vi "calibrateSteps.vi"(8 "error out":errorcluster, 9 "Direction":dbl, 10 "controllerAddress":i32, 11 "reference out":refnum<k24>) -> (0 "error out 2":errorcluster, 1 "mmPerStep":dbl, 2 "controllerAddress out":i32, 3 "reference out 2":refnum<k24>)   [LabVIEW 2013]
uses:
  C:/Program Files/Newport/Piezo Motion Control/Newport AG-UC2-UC8 Applet/Samples/LabVIEW 2009/AgilisCmdLib.dll
  Program Files/Newport/Piezo Motion Control/Newport AG-UC2-UC8 Applet/Samples/LabVIEW 2009/AgilisCmdLib.dll
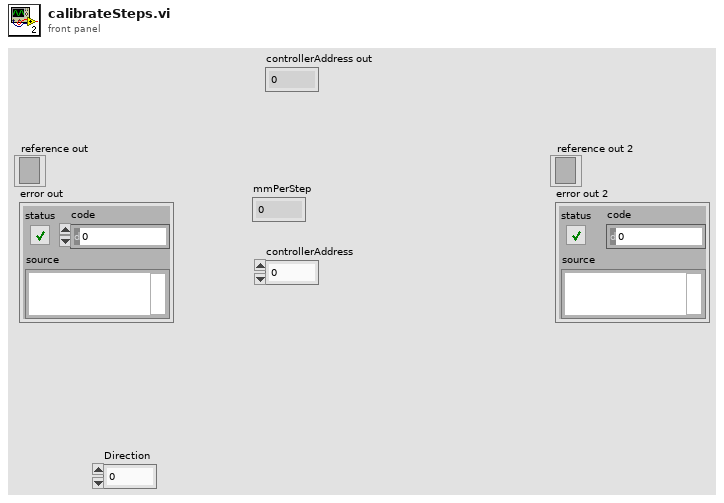
[diagram p1: front panel]
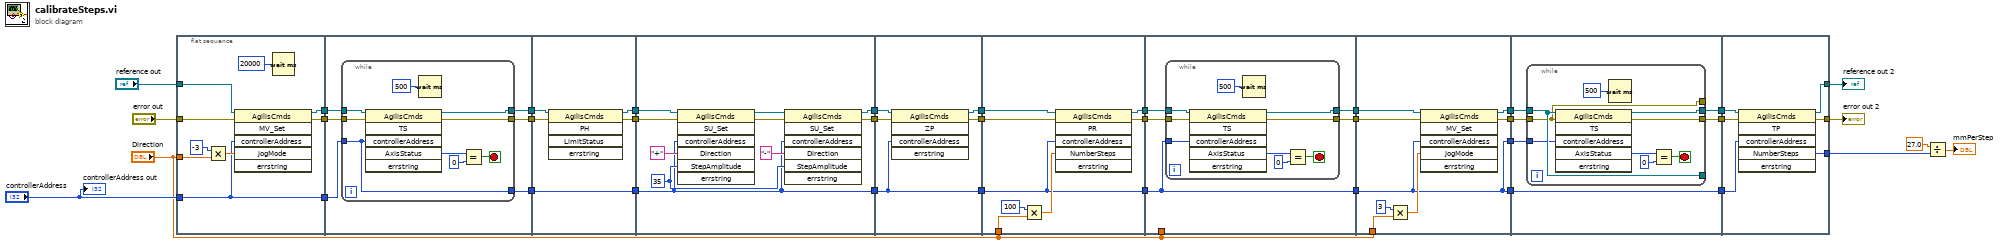
[diagram p0: block diagram]
diagram:
  n1 = flat-sequence {
    tunnel: "Direction" -> [w39]
    tunnel: "controllerAddress" -> [w40]
    tunnel: "error out" -> [w43]
    tunnel: "reference out" -> [w44]
    tunnel: [w42] -> w21
    tunnel: [w41] -> w20
    tunnel: [w40] -> w17
    tunnel: [w52] -> w37
    tunnel: [w51] -> w36
    tunnel: w21 -> [w50]
    tunnel: w20 -> [w49]
    tunnel: w17 -> [w48]
    tunnel: [w47] -> w15
    tunnel: w37 -> [w66]
    tunnel: w36 -> [w63]
    tunnel: [w65] -> w35
    tunnel: [w64] -> w34
    tunnel: [w62] -> w16
    tunnel: w15 -> [w62]
    tunnel: w35 -> [w75]
    tunnel: w34 -> [w74]
    tunnel: [w70] -> w33
    tunnel: [w72] -> w32
    tunnel: w16 -> [w67]
    tunnel: [w67] -> w14
    tunnel: w33 -> [w81]
    tunnel: w32 -> [w80]
    tunnel: [w79] -> w19
    tunnel: [w78] -> w18
    tunnel: w14 -> [w77]
    tunnel: [w77] -> w13
    tunnel: w19 -> [w87]
    tunnel: w18 -> [w86]
    tunnel: w13 -> [w85]
    tunnel: [w85] -> w12
    tunnel: [w84] -> w11
    tunnel: [w83] -> w10
    tunnel: "Direction" -> [w82]
    tunnel: [w94] -> w31
    tunnel: [w93] -> w30
    tunnel: "Direction" -> [_]
    tunnel: w12 -> [w90]
    tunnel: w11 -> [w92]
    tunnel: w10 -> [w91]
    tunnel: [w90] -> w7
    tunnel: w31 -> [w111]
    tunnel: w30 -> [w110]
    tunnel: "Direction" -> [w108]
    tunnel: [w106] -> w9
    tunnel: [w105] -> w8
    tunnel: w7 -> [w104]
    tunnel: [w104] -> w6
    tunnel: [w104] -> w5
    tunnel: w9 -> [w117]
    tunnel: w8 -> [w116]
    tunnel: w6 -> [w115]
    tunnel: w5 -> [w114]
    tunnel: [w114] -> w4
    tunnel: [w113] -> w3
    tunnel: [w112] -> w2
    tunnel: [w131] -> w26
    tunnel: [w132] -> w27
    tunnel: [w130] -> w24
    tunnel: w4 -> [w129]
    tunnel: w3 -> [w128]
    tunnel: w2 -> [w127]
    frame #0 {
      n2 = Multiply(x=-3 ("JogMode"), y=w39) -> (x*y=w46:dbl)
      n3 = invoke class="AgilisCmds" method="MV_Set"(reference=w44, error in=w43, "controllerAddress"=w40, "JogMode"=w46) -> (reference out=w42:refnum<k24>, error out=w41:errorcluster)  [unwired: 2 in, 4 out]
      n4 = Wait (ms)(milliseconds to wait=u32 20000) -> ()  [unwired: 1 out]
    }
    frame #1 {
      n5 = while {
        tunnel: [w61] -> w51
        tunnel: [w56] -> w52
        tunnel: w50 -> [w55]
        tunnel: w49 -> [w54]
        tunnel: w48 -> [w53]
        tunnel: [w53] -> w47
        stop <- w58 stop-if-true
        n6 = invoke class="AgilisCmds" method="TS"(reference=w55, error in=w54, "controllerAddress"=w53) -> (reference out=w56:refnum<k24>, error out=w61:errorcluster, "AxisStatus"=w60:i32)  [unwired: 3 in, 3 out]
        n7 = Wait (ms)(milliseconds to wait=u32 500) -> ()  [unwired: 1 out]
        n8 = Equal?(x=w60, y=0) -> (x = y?=w58:bool)
      }
    }
    frame #2 {
      n9 = invoke class="AgilisCmds" method="PH"(reference=w66, error in=w63) -> (reference out=w65:refnum<k24>, error out=w64:errorcluster)  [unwired: 3 in, 3 out]
    }
    frame #3 {
      w68 = 35 ("StepAmplitude")
      n10 = invoke class="AgilisCmds" method="SU_Set"(reference=w75, error in=w74, "controllerAddress"=w67, "Direction"="+", "StepAmplitude"=w68) -> (reference out=w71:refnum<k24>, error out=w73:errorcluster)  [unwired: 2 in, 5 out]
      n11 = invoke class="AgilisCmds" method="SU_Set"(reference=w71, error in=w73, "controllerAddress"=w67, "Direction"="-" ("Direction 2"), "StepAmplitude"=w68) -> (reference out=w70:refnum<k24>, error out=w72:errorcluster)  [unwired: 2 in, 5 out]
    }
    frame #4 {
      n12 = invoke class="AgilisCmds" method="ZP"(reference=w81, error in=w80, "controllerAddress"=w77) -> (reference out=w79:refnum<k24>, error out=w78:errorcluster)  [unwired: 2 in, 3 out]
    }
    frame #5 {
      n13 = Multiply(x=i64 100 ("NumberSteps"), y=w82) -> (x*y=w88:dbl)
      n14 = invoke class="AgilisCmds" method="PR"(reference=w87, error in=w86, "controllerAddress"=w85, "NumberSteps"=w88) -> (reference out=w84:refnum<k24>, error out=w83:errorcluster)  [unwired: 2 in, 4 out]
    }
    frame #6 {
      n15 = while {
        tunnel: [w103] -> w93
        tunnel: [w98] -> w94
        tunnel: w90 -> [w97]
        tunnel: w92 -> [w96]
        tunnel: w91 -> [w95]
        stop <- w100 stop-if-true
        n16 = invoke class="AgilisCmds" method="TS"(reference=w96, error in=w95, "controllerAddress"=w97) -> (reference out=w98:refnum<k24>, error out=w103:errorcluster, "AxisStatus"=w102:i32)  [unwired: 3 in, 3 out]
        n17 = Wait (ms)(milliseconds to wait=u32 500) -> ()  [unwired: 1 out]
        n18 = Equal?(x=w102, y=0) -> (x = y?=w100:bool)
      }
    }
    frame #7 {
      n19 = Multiply(x=3 ("JogMode 2"), y=w108) -> (x*y=w107:dbl)
      n20 = invoke class="AgilisCmds" method="MV_Set"(reference=w111, error in=w110, "controllerAddress"=w104, "JogMode"=w107) -> (reference out=w106:refnum<k24>, error out=w105:errorcluster)  [unwired: 2 in, 4 out]
    }
    frame #8 {
      n21 = while {
        tunnel: [w126] -> w112
        tunnel: [w120] -> _
        tunnel: [w119] -> _
        tunnel: [w121] -> w113
        tunnel: w117 -> [w120]
        tunnel: w116 -> [w119]
        tunnel: w115 -> [w118]
        stop <- w123 stop-if-true
        n22 = invoke class="AgilisCmds" method="TS"(reference=w120, error in=w119, "controllerAddress"=w118) -> (reference out=w121:refnum<k24>, error out=w126:errorcluster, "AxisStatus"=w125:i32)  [unwired: 3 in, 3 out]
        n23 = Wait (ms)(milliseconds to wait=u32 500) -> ()  [unwired: 1 out]
        n24 = Equal?(x=w125, y=0) -> (x = y?=w123:bool)
      }
    }
    frame #9 {
      n25 = invoke class="AgilisCmds" method="TP"(reference=w128, error in=w127, "controllerAddress"=w129) -> (reference out=w132:refnum<k24>, error out=w131:errorcluster, "NumberSteps"=w130:i32)  [unwired: 3 in, 3 out]
    }
  }
  n26 = Divide(x=27.0, y=w24) -> (x/y=→"mmPerStep":dbl)
  "reference out 2" <- w27
  "error out 2" <- w26
  "controllerAddress out" <- "controllerAddress"
